vi "MAVLink Message to Packet.vi"(8 "Error In":errorcluster, 11 "Message":string) -> (0 "Error Out":errorcluster, 3 "Packet":T1)   [LabVIEW 2014]
uses:
  Controls/MAVLink Packet.ctl
panel:
  out "Payload Length":u8
  out "Packet Sequence":u8 format="%x"
  out "System ID":u8
  out "Component ID":u8
  out "Message ID":u8
  out "Checksum":u16 format="%x"
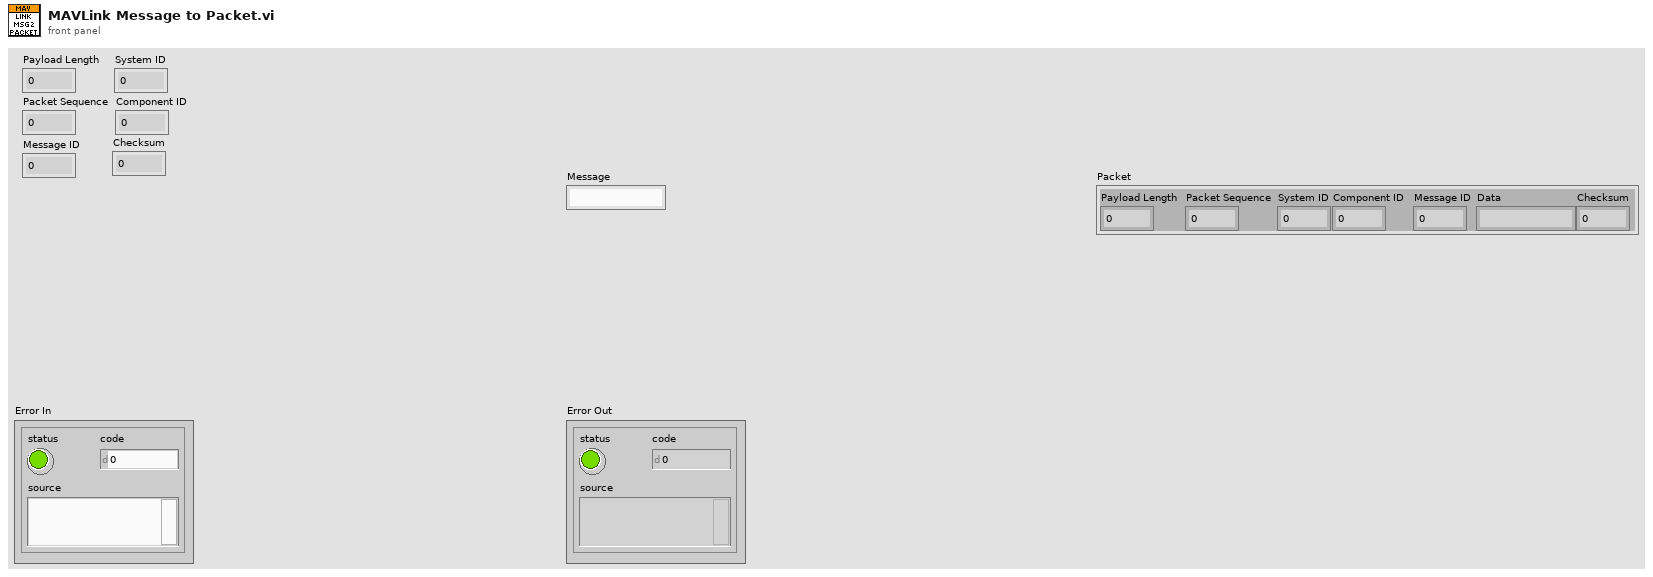
[diagram p1: front panel]
types:
  T1 = typedef "MAVLink Packet.ctl" = cluster{"Payload Length":u8, "Packet Sequence":u8, "System ID":u8, "Component ID":u8, "Message ID":u8, "Data":string, "Checksum":u16}
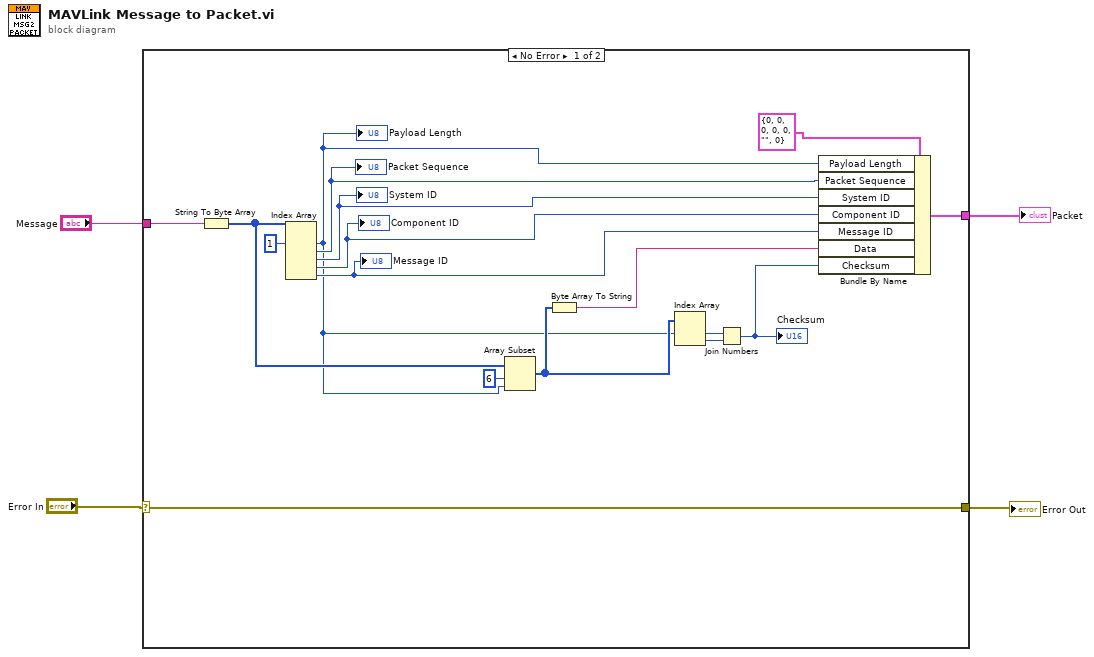
[diagram p0: block diagram]
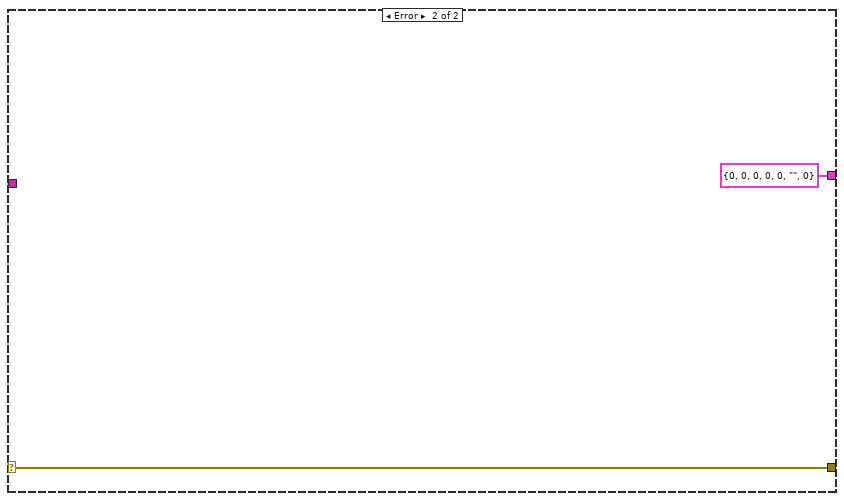
[diagram p2: hidden frame]
diagram:
  n1 = case shown="No Error" "Error In" {
    selector: "Error In" -> [w5 w22]
    tunnel: "Message" -> [w13 _]
    tunnel: [w12 T1 {"Payload Length"=0, "Packet Sequence"=0, "System ID"=0, "Component ID"=0, "Message ID"=0, "Data"="", "Checksum"=0} ("MAVLink Packet")] -> w3
    tunnel: [w5 w22] -> w1
    frame No Error {
      n2 = String To Byte Array(string=w13) -> (unsigned byte array=w7:u8[])
      n3 = Index Array(array=w7, index #1=1 ("index")) -> (element #1=w6:u8, element #2=w18:u8, element #3=w19:u8, element #4=w20:u8, element #5=w15:u8)  [unwired: 4 in]
      "Payload Length" <- w6
      "Packet Sequence" <- w18
      "System ID" <- w19
      "Component ID" <- w20
      "Message ID" <- w15
      n4 = Array Subset(array=w7, index=6, length=w6) -> (w9:u8[])
      n5 = Byte Array To String(unsigned byte array=w9) -> (string=w8:string)
      n6 = Index Array(array=w9, index #1=w6) -> (element #1=w17:u8, element #2=w16:u8)  [unwired: 1 in]
      n7 = Join Numbers(hi=w17, lo=w16) -> ((hi.lo)=w21:u16)
      "Checksum" <- w21
      n8 = Bundle By Name(cluster=T1 {"Payload Length"=0, "Packet Sequence"=0, "System ID"=0, "Component ID"=0, "Message ID"=0, "Data"="", "Checksum"=0} ("MAVLink Packet"), "Payload Length"=w6, "Packet Sequence"=w18, "System ID"=w19, "Component ID"=w20, "Message ID"=w15, "Data"=w8, "Checksum"=w21) -> (w12:T1)
    }
    frame Error {
    }
  }
  "Packet" <- w3
  "Error Out" <- w1
